vi "rqcBob Close.vi"(0 "rqcBob in":refnum<class "rqcBob.lvclass">, 11 "error in":errorcluster) -> (15 "error out":errorcluster)   [LabVIEW 2018, in "rqcBob.lvclass"]
uses:
  rqcBob.lvclass
  rqcBob.lvclass/rqcBob.ctl
  <vilib>/FPGAPlugInAG/Dynamic/niLvFpga_Close_Dynamic.vi
  <vilib>/rvi/interface/nirviCloseFPGA/nirviCloseFPGA.xnode
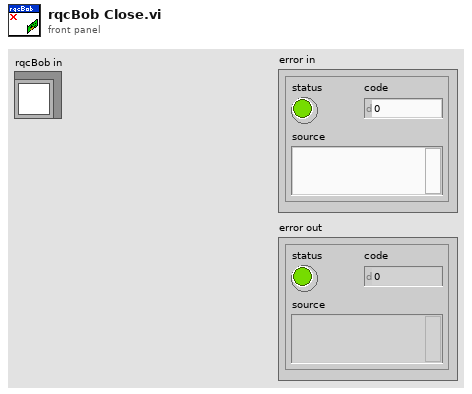
[diagram p1: front panel]
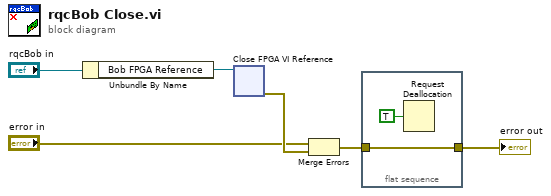
[diagram p0: block diagram]
diagram:
  n1 = Unbundle By Name("rqcBob in") -> ("Bob FPGA Reference"=w5:refnum<k20>)
  n2 = xnode "Close FPGA VI Reference"("FPGA VI Reference In"=w5) -> ("error out"=w4:errorcluster)  [unwired: 1 in]
  n3 = Merge Errors("error in", w4) -> (w2:errorcluster)
  n4 = flat-sequence {
    tunnel: [w8] -> w1
    tunnel: w2 -> [w8]
    frame #0 {
      n5 = Request Deallocation(TRUE ("flag")) -> ()
    }
  }
  "error out" <- w1
